vi "Omni Robot Body Model.vi"(10 "reset":bool, 11 "ccw torques":dbl[](array[numeric])=[1.0, 1.0, 1.0]) -> (0 "theta 2":dbl, 1 "x,y (inertial)":dbl[](array[numeric])=[0.0, 200.0], 2 "theta'":dbl, 3 "x',y' (inertial)":dbl[](array[numeric])=[0.0, 200.0], 4 "ccw wheel angles":dbl[](array[numeric]), 5 "ccw wheel angular velocities":dbl[](array[numeric]))   [LabVIEW 2015]
uses:
  <vilib>/Simulation/Implementation/Shared/SIMSCR Execution Mode.ctl
  <vilib>/Simulation/Scripting/Companion Diagram/SimConfigNode/SimParams.ctl
  <vilib>/Simulation/Scripting/Companion Diagram/SimConfigNode/_simSolvers.ctl
  <vilib>/Simulation/Param Hierarchy/Typedefs/SIMPH Param Control Actions.ctl
  <vilib>/Simulation/Implementation/Shared/SIM limit type.ctl
  <vilib>/Simulation/Implementation/Shared/NILVSim_ParamChanged.vi
  <vilib>/Simulation/Implementation/Shared/NILVSIM_BeginStep.vi
  <vilib>/Analysis/baseanly.llb/A x Vector.vi
  <vilib>/Simulation/ContinuousLinear/Implementation/NILVSim Integrator new.llb/SIM Integrator distributor (scalar).vi
  <vilib>/Simulation/ContinuousLinear/Implementation/NILVSim Integrator new.llb/SIM Integrator collector (scalar).vi
  <vilib>/Analysis/coordinate.llb/2D Cartesian Coordinate Rotation (Scalar).vi
  <vilib>/Simulation/ContinuousLinear/Implementation/NILVSim Integrator new.llb/SIM Integrator Distributor (vector).vi
  <vilib>/Simulation/ContinuousLinear/Implementation/NILVSim Integrator new.llb/SIM Integrator Collector (vector).vi
  <vilib>/Simulation/Implementation/Shared/NILVSim_Manager.vi
  <vilib>/Utility/error.llb/Clear Errors.vi
  <vilib>/Simulation/Implementation/Shared/NILVSim_FinalizeModel.vi
  <vilib>/Simulation/Implementation/Shared/SIM Unbundle Sim Info.vi
  <vilib>/Simulation/Implementation/Shared/SIMSH Read Queue.vi
  <vilib>/Simulation/Implementation/Shared/NILVSim_Initialize.vi
  <vilib>/Simulation/Utility/Implementation/NILVSim Get Time and IsAcceptedStep.vi
  <vilib>/Simulation/Implementation/Shared/NILVSim_GetModelError.vi
  <vilib>/Simulation/Implementation/Shared/SIM SimErrorHandler.vi
  <vilib>/Simulation/Implementation/Shared/SIM Bundle Sim Info.vi
  <vilib>/Simulation/Scripting/Companion Diagram/SimConfigNode/SimDog.xnode
  <vilib>/Analysis/NI_AALPro.lvlib
  <vilib>/Analysis/NI_AALBase.lvlib
  <vilib>/Simulation/Implementation/XNodeFramework/SimXNode/SimX.xnode
  <vilib>/Simulation/ContinuousLinear/Implementation/NILVSim Integrator new.llb/SIM Integrator (scalar).vi
  <vilib>/Simulation/ContinuousLinear/Implementation/NILVSim Integrator new.llb/SIM Integrator (vector).vi
  <vilib>/Simulation/Implementation/Shared/NI_SIM_Implementation.lvlib
panel:
  # "Motor Torques, in clockwise order from top left"
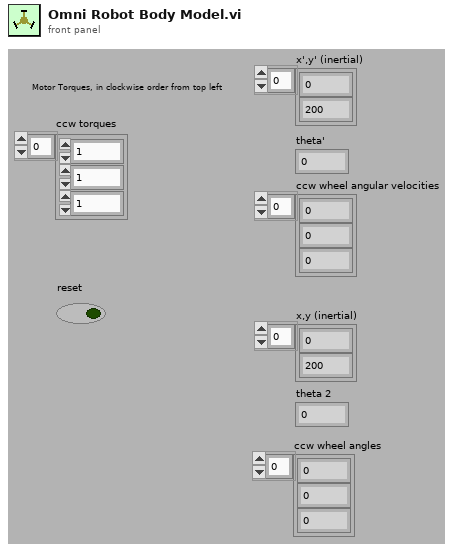
[diagram p1: front panel]
types:
  T1 = typedef "NI_Matrix.lvlib/RealMatrix.ctl" = dbl[][]
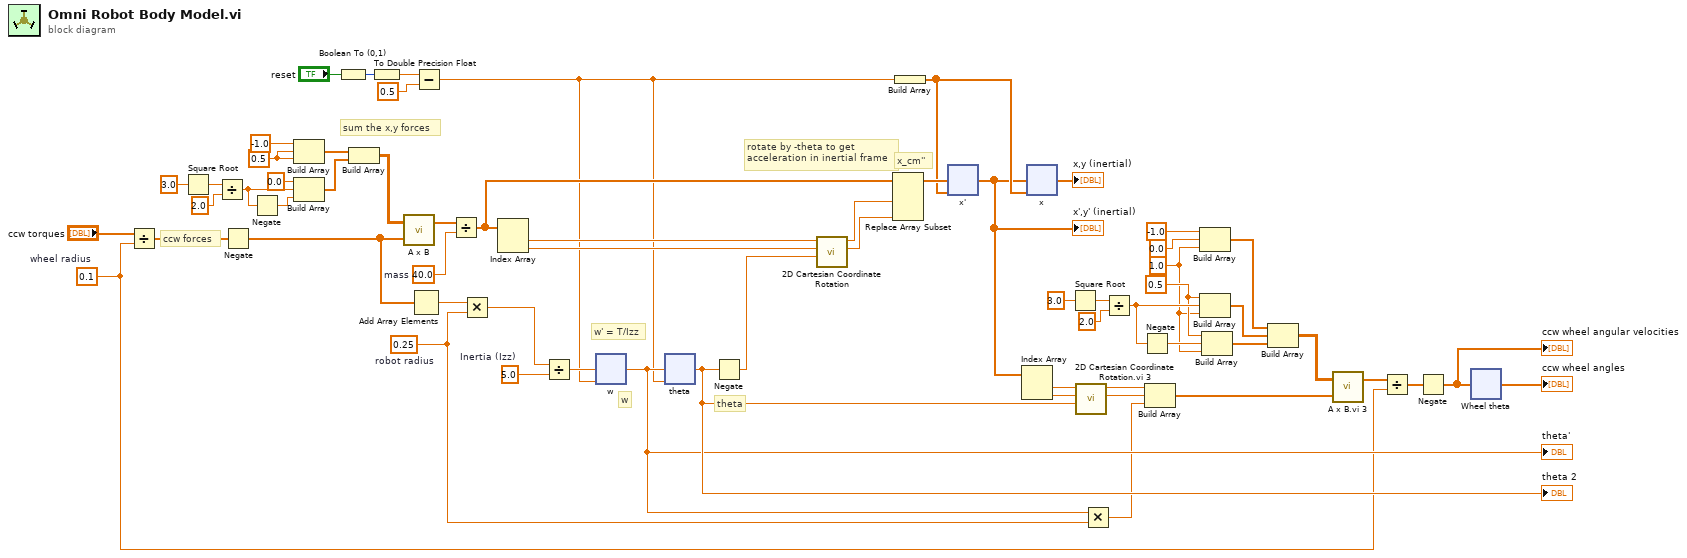
[diagram p0: block diagram]
diagram:
  w7 = 0.5 ("element")
  w5 = 1.0 ("element 7")
  w15 = 0.25  # robot radius
  w29 = 0.5 ("element 3")
  w48 = 5.0  # Inertia (Izz)
  w49 = 40.0  # mass
  w38 = 0.1  # wheel radius
  # "ccw forces"
  # "sum the x,y forces"
  # "x_cm''"
  # "rotate by -theta to get\nacceleration in inertial frame"
  # "theta"
  # "w"
  # "w' = T/Izz"
  n1 = Divide ("Divide 3")(x="ccw torques", y=w38) -> (x/y=w51:dbl[])
  n2 = Square Root(x=3.0 ("x 3")) -> (sqrt(x)=w27:dbl)
  n3 = Divide ("Divide 5")(x=w27, y=2.0 ("y 2")) -> (x/y=w24:dbl)
  n4 = Negate ("Negate 3")(x=w51) -> (-x=w18:dbl[])
  n5 = Negate ("Negate 2")(x=w24) -> (-x=w23:dbl)
  n6 = Build Array ("Build Array 3")(-1.0 ("element 2"), w29, w29) -> (w22:dbl[])
  n7 = Build Array ("Build Array 4")(0.0 ("element 4"), w24, w23) -> (w21:dbl[])
  n8 = Boolean To (0,1)(Boolean="reset") -> (0, 1=w35:i16)
  n9 = Build Array ("Build Matrix")(w22, w21) -> (w20:T1)
  n10 = To Double Precision Float(number=w35) -> (double precision float=w34:dbl)
  n11 = call-poly <vilib>:"A x B.vi"("Vector"=w18, "A"=w20) -> ("A x Vector"=w54:dbl[])  [unwired: 1 out]
  n12 = Add Array Elements(numeric array=w18) -> (sum=w17:dbl)
  n13 = Subtract(x=w34, y=0.5 ("x 2")) -> (x-y=w32:dbl)
  n14 = Divide ("Divide 2")(x=w54, y=w49) -> (x/y=w57:dbl[])
  n15 = Multiply ("Multiply 2")(x=w17, y=w15) -> (x*y=w16:dbl)
  n16 = Index Array(array=w57) -> (element #1=w61:dbl, element #2=w60:dbl)  [unwired: 2 in]
  n17 = Divide(x=w16, y=w48) -> (x/y=w62:dbl)
  n18 = xnode "w"("input"=w62, "reset"=w32) -> ("output"=w44:dbl)  [unwired: 8 in, 2 out]
  "theta'" <- w44
  n19 = xnode "theta"("input"=w44, "reset"=w32) -> ("output"=w45:dbl)  [unwired: 8 in, 2 out]
  "theta 2" <- w45
  n20 = Negate(x=w45) -> (-x=w50:dbl)
  n21 = call-poly <vilib>:"2D Cartesian Coordinate Rotation.vi"("theta"=w50, "y"=w60, "x"=w61) -> ("y out"=w58:dbl, "x out"=w59:dbl)  [unwired: 6 in, 1 out]
  n22 = Replace Array Subset(array=w57, new element #1=w59, new element #2=w58) -> (w56:dbl[])  [unwired: 2 in]
  n23 = Build Array ("Build Array 2")(w32) -> (w31:dbl[])
  n24 = xnode "x'"("input"=w56, "reset"=w31) -> ("output"=w19:dbl[])  [unwired: 8 in, 2 out]
  "x',y' (inertial)" <- w19
  n25 = Index Array ("Index Array 2")(array=w19) -> (element #1=w47:dbl, element #2=w46:dbl)  [unwired: 2 in]
  n26 = xnode "x"("input"=w19, "reset"=w31) -> ("output"=→"x,y (inertial)":dbl[])  [unwired: 8 in, 2 out]
  n27 = Square Root ("Square Root 2")(x=3.0 ("x 4")) -> (sqrt(x)=w10:dbl)
  n28 = call-poly "2D Cartesian Coordinate Rotation.vi 3"("theta"=w45, "y"=w46, "x"=w47) -> ("y out"=w41:dbl, "x out"=w42:dbl)  [unwired: 7 out]
  n29 = Multiply(x=w44, y=w15) -> (x*y=w43:dbl)
  n30 = Divide ("Divide 6")(x=w10, y=2.0) -> (x/y=w8:dbl)
  n31 = Negate ("Negate 4")(x=w8) -> (-x=w6:dbl)
  n32 = Build Array(w42, w41, w43) -> (w40:dbl[])
  n33 = Build Array ("Build Array 5")(-1.0 ("element 5"), 0.0 ("element 6"), w5) -> (w14:dbl[])
  n34 = Build Array ("Build Array 6")(w7, w8, w5) -> (w4:dbl[])
  n35 = Build Array ("Build Array 7")(w7, w6, w5) -> (w3:dbl[])
  n36 = Build Array ("Build Matrix 2")(w14, w4, w3) -> (w2:T1)
  n37 = call-poly "A x B.vi 3"("Vector"=w40, "A"=w2) -> ("A x Vector"=w39:dbl[])  [unwired: 1 out]
  n38 = Divide ("Divide 4")(x=w39, y=w38) -> (x/y=w37:dbl[])
  n39 = Negate ("Negate 5")(x=w37) -> (-x=w1:dbl[])
  "ccw wheel angular velocities" <- w1
  n40 = xnode "Wheel theta"("input"=w1) -> ("output"=→"ccw wheel angles":dbl[])  [unwired: 9 in, 2 out]
